vi "Cleanup VI FP.vi"(8 "error in":errorcluster, 11 "vi in":refnum<vi>) -> (0 "error out":errorcluster, 3 "vi out":refnum<vi>)   [LabVIEW 2019, in "gRPC Template Creation Utility.lvlib"]
uses:
  gRPC Template Creation Utility.lvlib
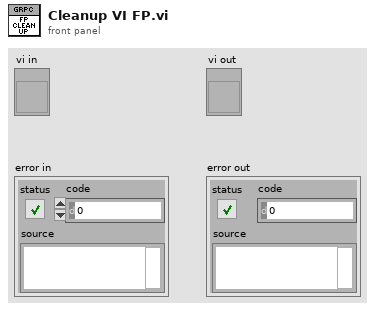
[diagram p1: front panel]
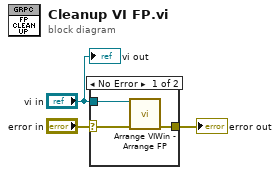
[diagram p0: block diagram]
diagram:
  n1 = case shown="No Error" "error in" {
    selector: "error in" -> [w4 w7]
    tunnel: [w6 w7] -> w3
    tunnel: "vi in" -> [w5 _]
    frame No Error {
      n2 = call <resource>:"Arrange VIWin - Arrange FP.vi"("VI"=w5, "error in"=w4) -> ("error out"=w6:errorcluster)  [unwired: 13 in]
    }
    frame Error {
    }
  }
  "error out" <- w3
  "vi out" <- "vi in"
